vi "Call_signal_fromHW.vi"(5 "Plot window":string) -> (1 "Selected signals":string[](array[string]), 2 "Ready?":bool)   [LabVIEW 2021]
doc: "Through this function you can select the stored signals from the Main_menu."
panel:
  in  "Working Path":path
  in  "Load Signals profile":bool
  in  "Save Signals profile":bool
  in  "Select signals":i32[](listbox)
  out "Clone Name":string
  in  "Add to graph":bool
  # "First Save Signals before\nto load Signals"
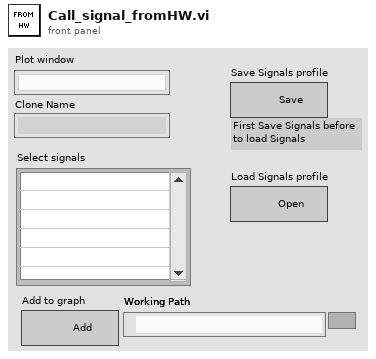
[diagram p1: front panel]
types:
  T1 = enum32{"Invalid", "Standard", "Closed", "Hidden", "Minimized", "Maximized"}
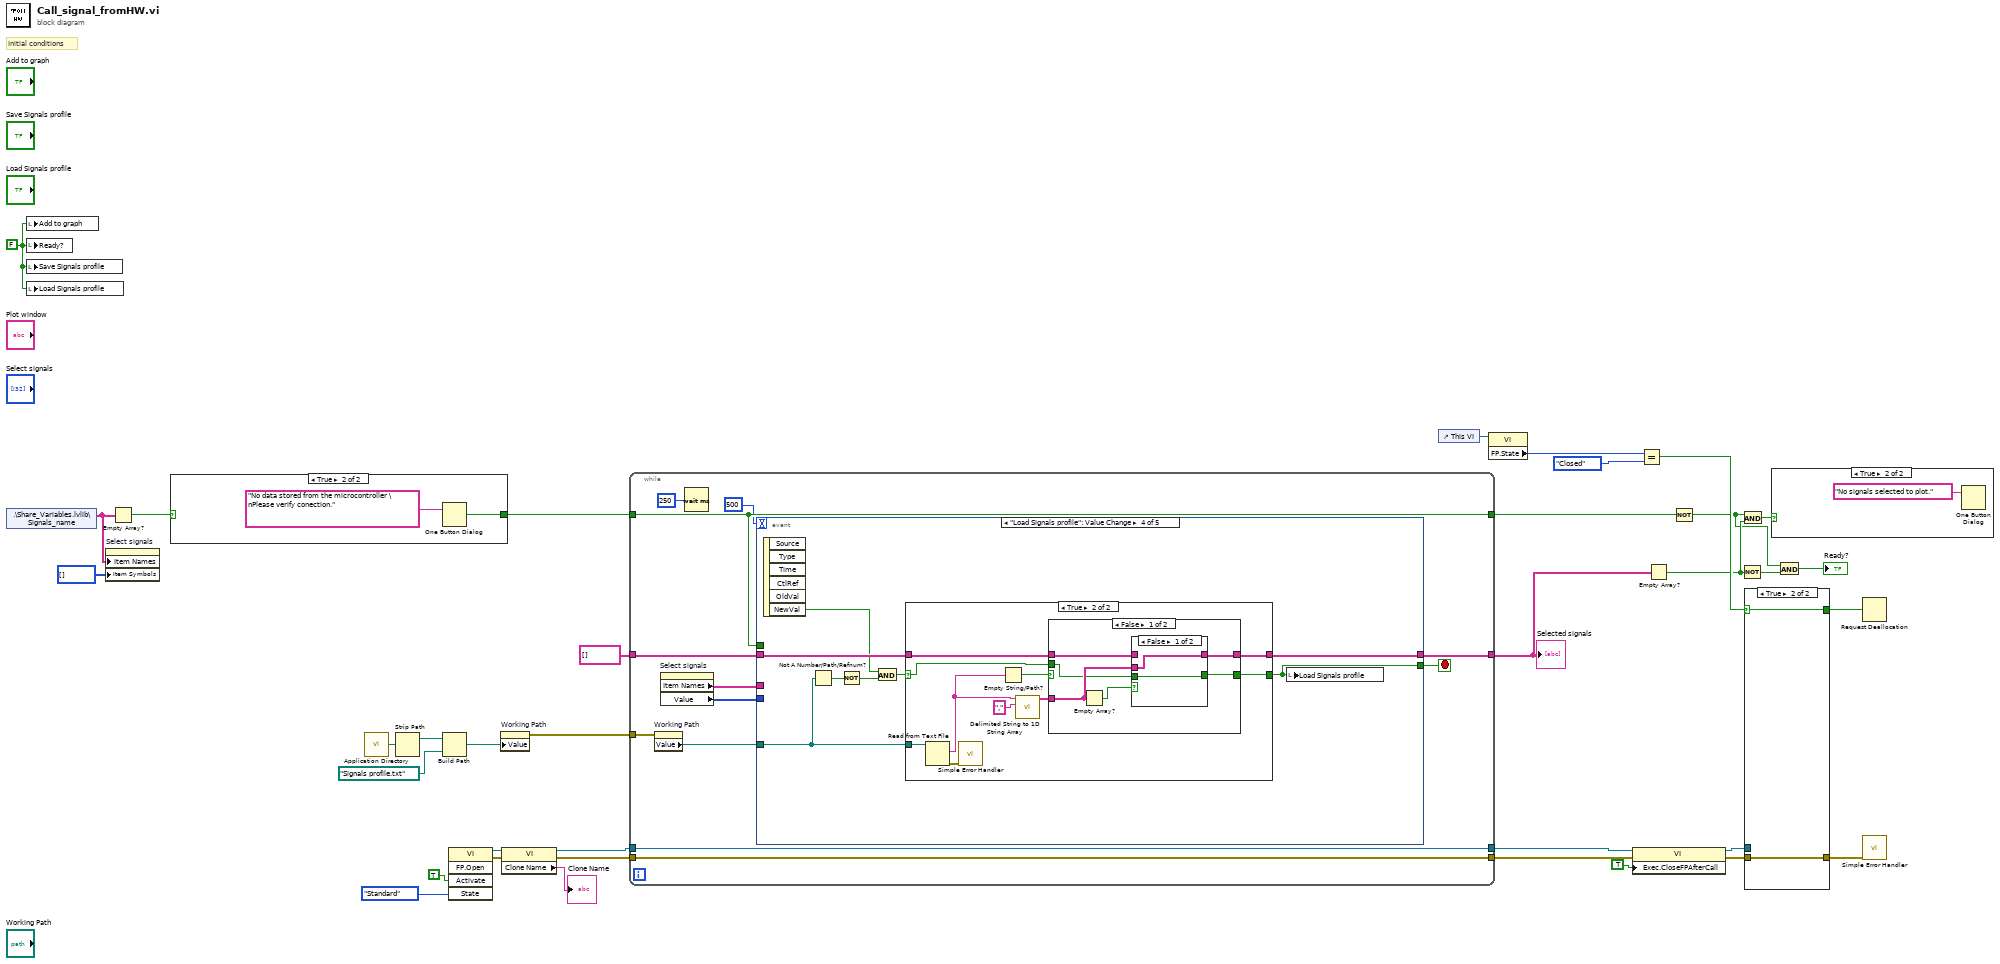
[diagram p0: block diagram]
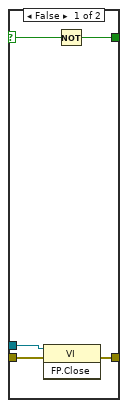
[diagram p2: hidden frame]
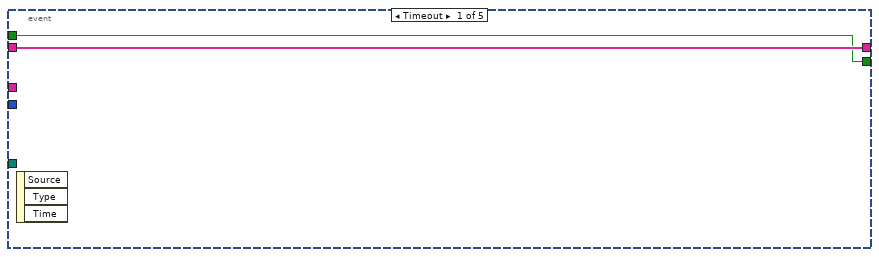
[diagram p5: hidden frame]
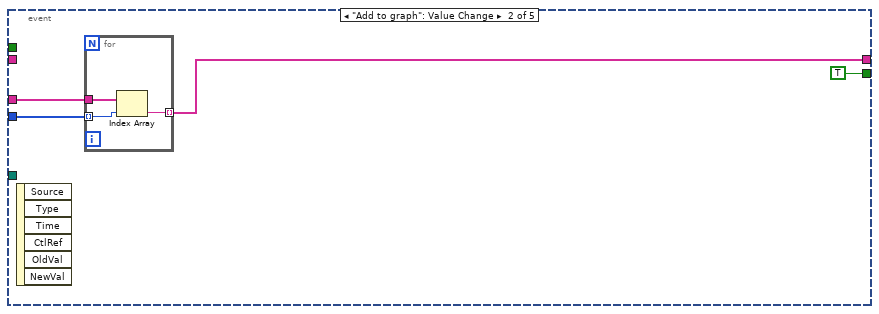
[diagram p6: hidden frame]
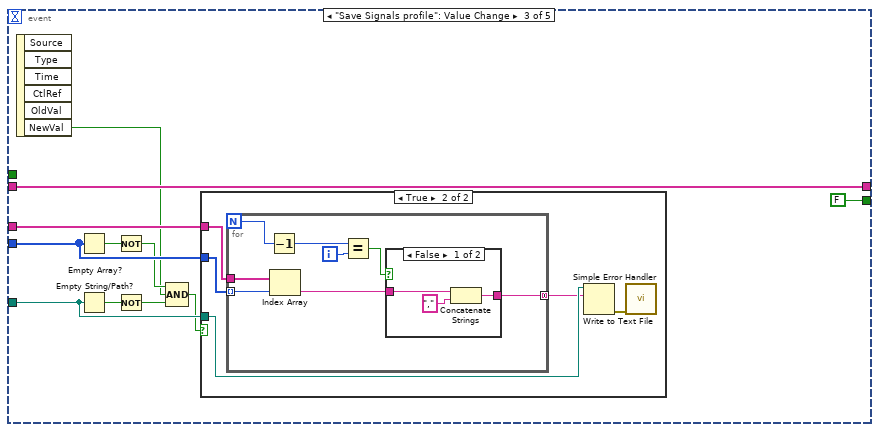
[diagram p7: hidden frame]
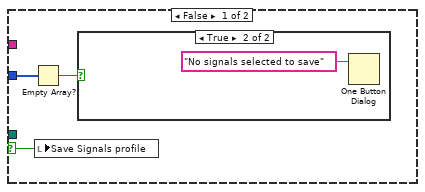
[diagram p8: hidden frame]
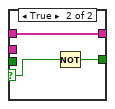
[diagram p12: hidden frame]
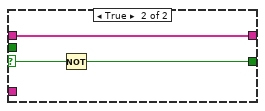
[diagram p13: hidden frame]
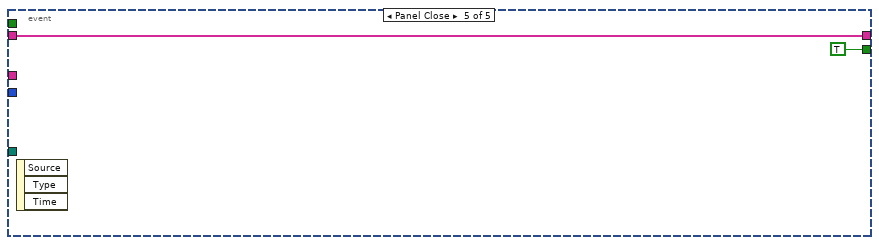
[diagram p14: hidden frame]
diagram:
  w19 = FALSE
  # "Initial conditions"
  n1 = shared-variable ".\\Share_Variables.lvlib\\Signals_name"() -> (w22:string[])  [unwired: 1 in, 1 out]
  n2 = local write "Add to graph"(w19) -> ()
  n3 = local write "Ready?"(w19) -> ()
  n4 = local write "Save Signals profile"(w19) -> ()
  n5 = local write "Load Signals profile"(w19) -> ()
  n6 = property on="Select signals" class="LstBox (strict)"("Item Names"=w22, "Item Symbols"=i32[] []) -> ()  [unwired: 2 in, 2 out]
  n7 = Empty Array?(array=w22) -> (empty?=w26:bool)
  n8 = case shown="True" w26 {
    selector: w26 -> [w37 _]
    tunnel: [w37 w38] -> w25
    frame False {
    }
    frame True {
      n9 = One Button Dialog(message="No data stored from the microcontroller \nPlease verify conection.") -> (true=w38:bool)  [unwired: 1 in]
    }
  }
  n10 = call <vilib>:"Application Directory.vi"() -> ("Application Directory"=w14:path)
  n11 = Strip Path(path=w14) -> (stripped path=w18:path)  [unwired: 1 out]
  n12 = Build Path(base path=w18, name or relative path=path "Signals profile.txt" ("default name")) -> (appended path=w2:path)
  n13 = invoke on="Invoke Node" class="VI" method="FP.Open"("Activate"=TRUE ("Activate?"), "State"=T1."Standard") -> (reference out=w33:refnum<vi>, error out=w34:errorcluster)  [unwired: 3 in, 3 out]
  n14 = property on="Working Path" class="Path"("Value"=w2) -> (error out=w1:errorcluster)  [unwired: 2 in, 1 out]
  n15 = property on="Property Node" class="VI"(reference=w33, error in=w34) -> (reference out=w32:refnum<vi>, error out=w35:errorcluster, "Clone Name"=→"Clone Name":string)
  n16 = while {
    tunnel: w35 -> [w51]
    tunnel: w32 -> [w50]
    tunnel: [w50] -> w30
    tunnel: [w51] -> w29
    tunnel: w25 -> [w45]
    tunnel: [w49] -> w6
    tunnel: string[] [] -> [w48]
    tunnel: [w45] -> w8
    tunnel: w1 -> [w42]
    stop <- w44 stop-if-true
    n17 = property on="Working Path" class="Path"(error in=w42) -> ("Value"=w41:path)  [unwired: 1 in, 2 out]
    n18 = property on="Select signals" class="LstBox (strict)"() -> ("Item Names"=w47:string[], "Value"=w46:i32[])  [unwired: 2 in, 2 out]
    n19 = Wait (ms)(milliseconds to wait=u32 250) -> ()  [unwired: 1 out]
    n20 = event shown="[3] \"Load Signals profile\": Value Change" {
      selector: _ -> [_ _ _ _ _]
      dyn-events: _ -> [_ _ _ _ _]
      timeout: 500 -> [_ _ _ _ _]
      tunnel: [w52 TRUE FALSE ("true") w99 TRUE] -> w44
      tunnel: [w53 w55 w69 w100 w127] -> w49
      tunnel: w48 -> [w53 _ w69 w98 w127]
      tunnel: w47 -> [_ w57 w70 _ _]
      tunnel: w46 -> [_ w56 w68 _ _]
      tunnel: w41 -> [_ _ w66 w97 _]
      tunnel: w45 -> [w52 _ _ _ _]
      event Timeout {
        n21 = event-data() -> ()  [unwired: 1 in, 3 out]
      }
      event "Add to graph": Value Change {
        n22 = event-data() -> ()  [unwired: 1 in, 6 out]
        n23 = for {
          tunnel: w56 -> [w60] mode=indexing
          tunnel: [w59] -> w55 mode=indexing
          tunnel: w57 -> [w58]
          n24 = Index Array(array=w58, index=w60) -> (element=w59:string)
        }
      }
      event "Save Signals profile": Value Change {
        n25 = event-data() -> ("NewVal"=w63:bool)  [unwired: 1 in, 5 out]
        n26 = Empty Array?(array=w68) -> (empty?=w67:bool)
        n27 = Empty String/Path?(string/path=w66) -> (empty?=w65:bool)
        n28 = Not(x=w67) -> (.not. x?=w64:bool)
        n29 = Not(x=w65) -> (.not. x?=w62:bool)
        n30 = Compound Arithmetic op=AND(w64, w63, w62) -> (w61:bool)
        n31 = case shown="True" w61 {
          selector: w61 -> [w72 _]
          tunnel: w70 -> [_ w77]
          tunnel: w68 -> [w74 w78]
          tunnel: w66 -> [_ w80]
          frame False {
            n32 = Empty Array?(array=w74) -> (empty?=w73:bool)
            n33 = local write "Save Signals profile"(w72) -> ()
            n34 = case shown="True" w73 {
              frame False {
              }
              frame True {
                n35 = One Button Dialog(message="No signals selected to save") -> ()  [unwired: 1 in, 1 out]
              }
            }
          }
          frame True {
            n36 = for {
              N -> [w86]
              tunnel: w78 -> [w88] mode=indexing
              tunnel: w77 -> [w87]
              tunnel: [w81] -> w76 mode=concatenating
              i -> [w84]
              n37 = Decrement(x=w86) -> (x-1=w85:i32)
              n38 = Index Array(array=w87, index=w88) -> (element=w82:string)
              n39 = Equal?(x=w85, y=w84) -> (x = y?=w83:bool)
              n40 = case shown="False" w83 {
                tunnel: w82 -> [w90 w92]
                tunnel: [w89 w92] -> w81
                frame False {
                  n41 = Concatenate Strings(w90, "," ("string")) -> (w89:string)
                }
                frame True {
                }
              }
            }
            n42 = Write to Text File(file (use dialog)=w80, text=w76) -> (error out=w79:errorcluster)  [unwired: 2 in, 2 out]
            n43 = call <vilib>:"Simple Error Handler.vi"("error in (no error)"=w79) -> ()  [unwired: 4 in, 5 out]
          }
        }
      }
      event "Load Signals profile": Value Change {
        n44 = event-data() -> ("NewVal"=w93:bool)  [unwired: 1 in, 5 out]
        n45 = Not A Number/Path/Refnum?(number/path/refnum=w97) -> (NaN/Path/Refnum?=w96:bool)
        n46 = Not(x=w96) -> (.not. x?=w95:bool)
        n47 = And(x=w93, y=w95) -> (x .and. y?=w94:bool)
        n48 = case shown="True" w94 {
          selector: w94 -> [w102 w107]
          tunnel: [w101 w109] -> w100
          tunnel: [w102 w106] -> w99
          tunnel: w98 -> [w101 w108]
          tunnel: w97 -> [_ w112]
          frame False {
          }
          frame True {
            n49 = Read from Text File(file (use dialog)=w112) -> (text=w104:string, error out=w111:errorcluster)  [unwired: 3 in, 2 out]
            n50 = call <vilib>:"Simple Error Handler.vi"("error in (no error)"=w111) -> ()  [unwired: 4 in, 5 out]
            n51 = Empty String/Path?(string/path=w104) -> (empty?=w110:bool)
            n52 = call <vilib>:"Delimited String to 1D String Array.vi"("delimiter"=",", "delimited string"=w104) -> ("string array"=w103:string[])  [unwired: 9 in]
            n53 = case shown="False" w110 {
              selector: w110 -> [_ w125]
              tunnel: [w116 w126] -> w109
              tunnel: w108 -> [w115 w126]
              tunnel: w107 -> [w113 _]
              tunnel: [w114 w124] -> w106
              tunnel: w103 -> [w117 _]
              frame False {
                n54 = Empty Array?(array=w117) -> (empty?=w118:bool)
                n55 = case shown="False" w118 {
                  selector: w118 -> [_ w121]
                  tunnel: w117 -> [w120 _]
                  tunnel: [w120 w123] -> w116
                  tunnel: w115 -> [_ w123]
                  tunnel: [w119 w122] -> w114
                  tunnel: w113 -> [w119 _]
                  frame False {
                  }
                  frame True {
                    n56 = Not(x=w121) -> (.not. x?=w122:bool)
                  }
                }
              }
              frame True {
                n57 = Not(x=w125) -> (.not. x?=w124:bool)
              }
            }
          }
        }
        n58 = local write "Load Signals profile"(w99) -> ()
      }
      event Panel Close {
        n59 = event-data() -> ()  [unwired: 1 in, 3 out]
      }
    }
  }
  "Selected signals" <- w6
  n60 = control-ref of="This VI"() -> (w11:refnum<vi>)
  n61 = property class="VI"(reference=w11) -> ("FP.State"=w12:T1)  [unwired: 1 in, 2 out]
  n62 = property class="VI"(reference=w30, error in=w29, "Exec.CloseFPAfterCall"=TRUE ("Activate?")) -> (reference out=w28:refnum<vi>, error out=w27:errorcluster)
  n63 = Equal?(x=w12, y=T1."Closed" ("Front Panel Window:State")) -> (x = y?=w9:bool)
  n64 = Empty Array?(array=w6) -> (empty?=w5:bool)
  n65 = Not(x=w8) -> (.not. x?=w4:bool)
  n66 = Not(x=w5) -> (.not. x?=w7:bool)
  n67 = And(x=w4, y=w5) -> (x .and. y?=w3:bool)
  n68 = case shown="True" w9 {
    selector: w9 -> [w130 w134]
    tunnel: [w133 w135] -> w16
    tunnel: w28 -> [w132 _]
    tunnel: w27 -> [w131 w135]
    tunnel: [w129 w134] -> w15
    frame False {
      n69 = invoke class="VI" method="FP.Close"(reference=w132, error in=w131) -> (error out=w133:errorcluster)  [unwired: 1 in, 2 out]
      n70 = Not(x=w130) -> (.not. x?=w129:bool)
    }
    frame True {
    }
  }
  n71 = case shown="True" w3 {
    frame False {
    }
    frame True {
      n72 = One Button Dialog(message="No signals selected to plot.") -> ()  [unwired: 1 in, 1 out]
    }
  }
  n73 = And(x=w4, y=w7) -> (x .and. y?=→"Ready?":bool)
  n74 = Request Deallocation(w15) -> ()
  n75 = call <vilib>:"Simple Error Handler.vi"("error in (no error)"=w16) -> ()  [unwired: 4 in, 5 out]
